vi "Alarm interface.vi"(8 "错误输入（无错误）":errorcluster, 11 "簇":T1) -> (0 "错误输出":errorcluster)   [LabVIEW 2022 SP3, in "Alarm interface.lvlib"]
uses:
  Alarm interface.lvlib
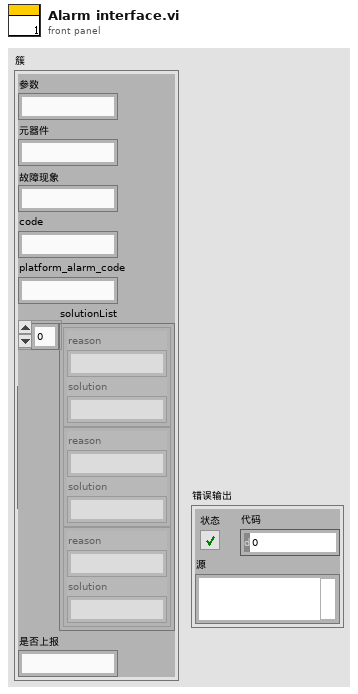
[diagram p1: front panel]
types:
  T1 = typedef "Alarm interface.lvlib/报警短信语音交互.ctl" = cluster{"参数":string, "元器件":string, "故障现象":string, "code":string, "platform_alarm_code":string, "solutionList":cluster{"reason":string, "solution":string}[], "是否上报":string}
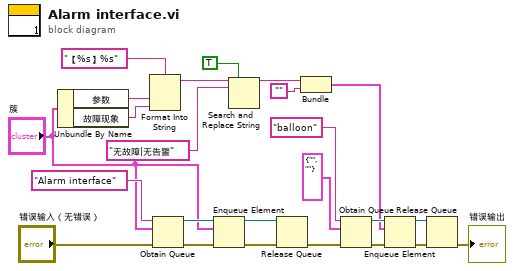
[diagram p0: block diagram]
diagram:
  n1 = Unbundle By Name("簇") -> ("参数"=w14:string, "故障现象"=w7:string)
  n2 = Format Into String(format string="【%s】%s" ("格式字符串"), w14, w7) -> (resulting string=w9:string)  [unwired: 2 in, 1 out]
  n3 = Obtain Queue(name (unnamed)="Alarm interface" ("名称（未命名）"), element data type="簇", error in (no error)="错误输入（无错误）") -> (queue out=w21:refnum<queue>, error out=w22:errorcluster)  [unwired: 2 in, 1 out]
  n4 = Enqueue Element(queue=w21, element="簇", error in (no error)=w22) -> (queue out=w23:refnum<queue>, error out=w24:errorcluster)  [unwired: 1 in, 1 out]
  n5 = Search and Replace String(replace all?=TRUE ("替换全部？(F)"), input string=w9, search string="无故障|无告警" ("字符串")) -> (result string=w12:string)  [unwired: 5 in, 3 out]
  n6 = Release Queue(queue=w23, error in (no error)=w24) -> (error out=w4:errorcluster)  [unwired: 1 in, 2 out]
  n7 = Bundle("result string"=w12, "") -> (w2:cluster{"result string":string, string})  [unwired: 1 in]
  n8 = Obtain Queue(name (unnamed)="balloon" ("名称（未命名）"), element data type=cluster{"Title":string, "Body":string} {"Title"="", "Body"=""}, error in (no error)=w4) -> (queue out=w13:refnum<queue>, error out=w8:errorcluster)  [unwired: 2 in, 1 out]
  n9 = Enqueue Element(queue=w13, element=w2, error in (no error)=w8) -> (queue out=w6:refnum<queue>, error out=w5:errorcluster)  [unwired: 1 in, 1 out]
  n10 = Release Queue(queue=w6, error in (no error)=w5) -> (error out=→"错误输出":errorcluster)  [unwired: 1 in, 2 out]
